vi "Lidar Mapping.vi"(4 "Center y":dbl, 5 "grid dimension y":i32, 6 "Center x":dbl, 7 "grid dimension x":i32, 10 "Distance to Obstacles":dbl, 11 "Heading":dbl(knob) scale=-90.0..90.0) -> (3 "Occupancy Grid Instance 2":dbl[][](graph))   [LabVIEW 2015]
uses:
  <vilib>/Analysis/coordinate.llb/2D Cartesian Coordinate Rotation (Array).vi
  <vilib>/Analysis/NI_AALPro.lvlib
panel:
  out "y":dbl=50.0
  out "x":dbl=50.0
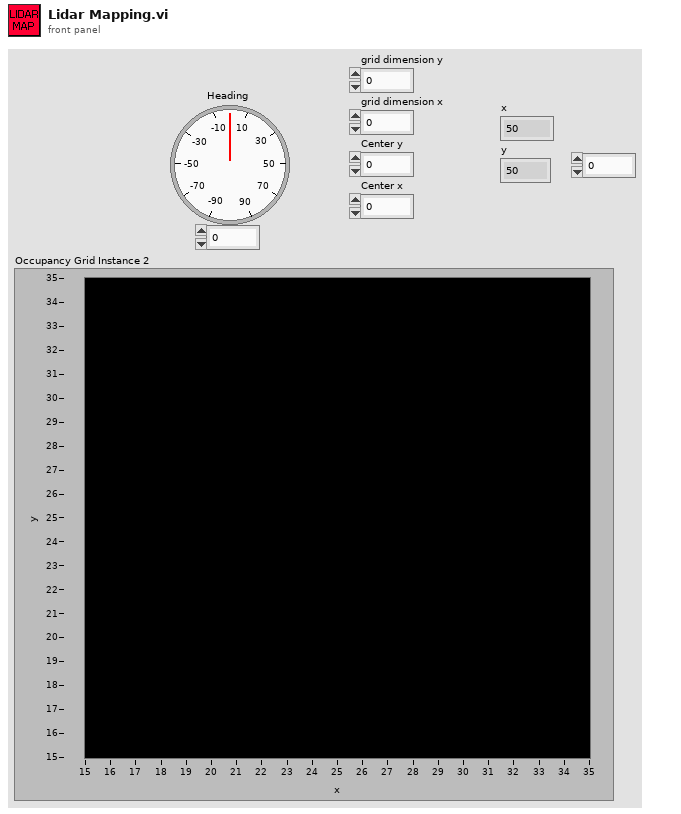
[diagram p1: front panel]
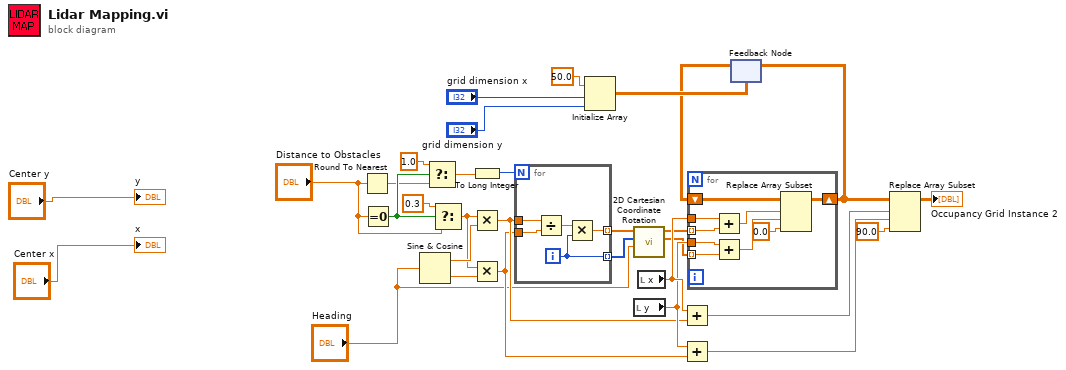
[diagram p0: block diagram]
diagram:
  n1 = Round To Nearest(number="Distance to Obstacles") -> (nearest integer value=w21:dbl)
  n2 = Equal To 0?(x="Distance to Obstacles") -> (x = 0?=w23:bool)
  n3 = Sine & Cosine(0:"Heading") -> (1:w30:dbl, 2:w29:dbl)
  n4 = Select(t=1.0, s=w23, f=w21) -> (s? t:f=w22:dbl)
  n5 = Select(t=0.3, s=w23, f="Distance to Obstacles") -> (s? t:f=w25:dbl)
  n6 = To Long Integer(number=w22) -> (32bit integer=w19:i32)
  n7 = Multiply(x=w25, y=w30) -> (x*y=w12:dbl)
  n8 = Multiply(x=w25, y=w29) -> (x*y=w11:dbl)
  n9 = for {
    N: w19 -> [_]
    tunnel: w12 -> [w35]
    tunnel: w11 -> [w34]
    tunnel: [w33] -> w16 mode=indexing
    tunnel: [w32] -> w15 mode=indexing
    i -> [w32]
    n10 = Divide(x=w35, y=w34) -> (x/y=w36:dbl)
    n11 = Multiply(x=w36, y=w32) -> (x*y=w33:dbl)
  }
  n12 = Initialize Array(50.0 ("element"), "grid dimension x", "grid dimension y") -> (w3:dbl[][])
  n13 = call-poly <vilib>:"2D Cartesian Coordinate Rotation.vi"("theta"="Heading", "Y"=w15, "X"=w16) -> ("Y Out"=w14:dbl[], "X Out"=w13:dbl[])  [unwired: 6 in, 1 out]
  n14 = local read "y"() -> (w27:dbl)
  n15 = local read "x"() -> (w28:dbl)
  n16 = Add(x=w28, y=w12) -> (x+y=w17:dbl)
  n17 = Add(x=w27, y=w11) -> (x+y=w18:dbl)
  n18 = feedback #1(w3) -> (w2:dbl[][])
  n19 = for {
    tunnel: w28 -> [w45]
    tunnel: w27 -> [w44]
    tunnel: w13 -> [w39] mode=indexing
    tunnel: w14 -> [w38] mode=indexing
    shift-right: [w42] -> w1
    shift-left: w2 -> [w43]
    n20 = Add(x=w45, y=w39) -> (x+y=w40:dbl)
    n21 = Add(x=w44, y=w38) -> (x+y=w41:dbl)
    n22 = Replace Array Subset(array=w43, new element=0.0 ("new element/subarray"), index (row)=w40, index (col)=w41) -> (w42:dbl[][])
  }
  n23 = feedback-in #1(w1) -> ()
  n24 = Replace Array Subset(array=w1, new element=90.0 ("new element/subarray"), index (row)=w17, index (col)=w18) -> (→"Occupancy Grid Instance 2":dbl[][])
  "x" <- "Center x"
  "y" <- "Center y"
